vi "LIMITSdll.vi"(8 "error in (no error)":errorcluster, 11 "Inputs":cluster{"htyp":string, "z":dbl[]}) -> (0 "error out":errorcluster, 3 "Outputs":T1)   [LabVIEW 2021]
doc: "subroutine LIMITSdll(htyp, z, tmin, tmax, dmax, pmax, htyp_length)\nReturns limits of a property model as a function of composition. Pure fluid limits were read in from the *.fld files; for mixtures, a simple mole fraction weighting in reduced variables is used.\n\nINPUTS:\nhtyp -- Flag indicating which models are to be checked (character*3) \n ‘EOS’: Equation of state for thermodynamic properties \n ‘ETA’: Viscosity \n ‘TCX’: Thermal conductivity\n ‘STN’: Surface tension\nz -- Composition array (array of mole fractions)\n\nOUTPUTS:\ntmin -- Minimum temperature for model specified by htyp [K]\ntmax -- Maximum temperature [K]\ndmax -- Maximum density [mol/L]\npmax -- Maximum pressure [kPa]\nhtyp_length -- length of variable htyp (default: 3)"
uses:
  REFPROP.dll
panel:
  # "REFPROP-LIMITSdll.vi"
  # "void  LIMITSdll(CStr htyp, double *z, double *tmin, double *tmax, double *dmax, double *pmax, int32_t *hyp_length);"
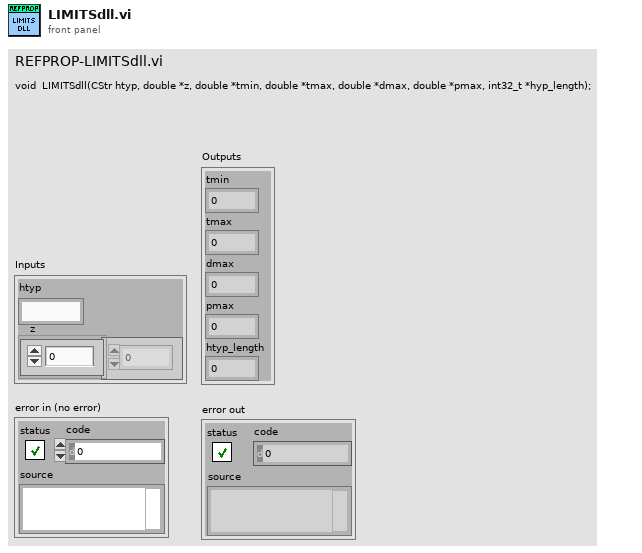
[diagram p1: front panel]
types:
  T1 = cluster{"tmin":dbl, "tmax":dbl, "dmax":dbl, "pmax":dbl, "htyp_length":i32}
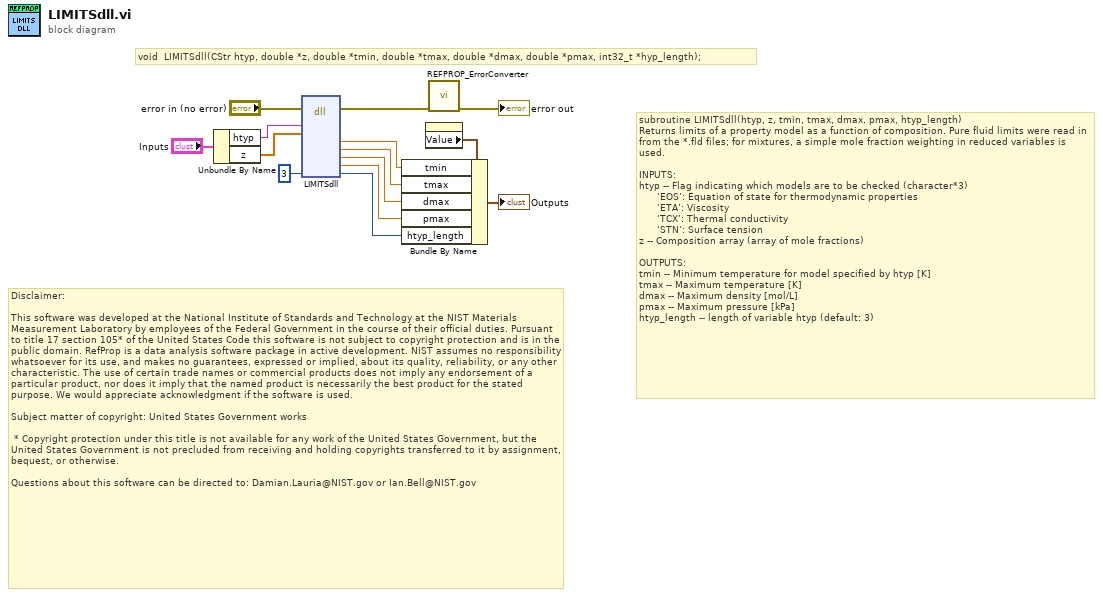
[diagram p0: block diagram]
diagram:
  # "Disclaimer:\n\nThis software was developed at the National Institute of Standards and Technology at the NIST Materials Measurement Laboratory by employees of the Federal Government in the course of their official duties. Pursuant to title 17 section 105* of the United States Code this software is not subject to copyright protection and is in the public domain. RefProp is a data analysis software package in active development. NIST assumes no responsibility whatsoever for its use, and makes no guarantees, expressed or implied, about its quality, reliability, or any other characteristic. The use of certain trade names or commercial products does not imply any endorsement of a particular product, nor does it imply that the named product is necessarily the best product for the stated purpose. We would appreciate acknowledgment if the software is used.\n \nSubject matter of copyright: United States Government works\n  \n * Copyright protection under this title is not available for any work of the United States Government, but the United States Government is not precluded from receiving and holding copyrights transferred to it by assignment, bequest, or otherwise.\n\nQuestions about this software can be directed to: Damian.Lauria@NIST.gov or Ian.Bell@NIST.gov"
  # "void  LIMITSdll(CStr htyp, double *z, double *tmin, double *tmax, double *dmax, double *pmax, int32_t *hyp_length);"
  # "subroutine LIMITSdll(htyp, z, tmin, tmax, dmax, pmax, htyp_length)\nReturns limits of a property model as a function of composition. Pure fluid limits were read in from the *.fld files; for mixtures, a simple mole fraction weighting in reduced variables is used.\n\nINPUTS:\nhtyp -- Flag indicating which models are to be checked (character*3) \n      ‘EOS’: Equation of state for thermodynamic properties \n      ‘ETA’: Viscosity \n      ‘TCX’: Thermal conductivity\n      ‘STN’: Surface tension\nz -- Composition array (array of mole fractions)\n\nOUTPUTS:\ntmin -- Minimum temperature for model specified by htyp [K]\ntmax -- Maximum temperature [K]\ndmax -- Maximum density [mol/L]\npmax -- Maximum pressure [kPa]\nhtyp_length -- length of variable htyp (default: 3)"
  n1 = Unbundle By Name("Inputs") -> ("htyp"=w9:string, "z"=w8:dbl[])
  n2 = dll-call lib="C:/Users/lauria/OneDrive - National Institute of Standards and Technology (NIST)/LabVIEW Projects/7 REFPROP/REFPROP-wrappers-master/REFPROP-wrappers-master/wrappers/Labview/REFPROP/REFPROP.*" fn="LIMITSdll"(error in="error in (no error)", "htyp"=w9, "z"=w8, "hyp_length"=3 ("ln")) -> (error out=w14:errorcluster, "tmin"=w1:dbl, "tmax"=w2:dbl, "dmax"=w3:dbl, "pmax"=w4:dbl, "hyp_length"=w5:i32)  [unwired: 9 in, 1 out]
  n3 = property on="Outputs" class="Clust (strict)"() -> ("Value"=w6:T1)  [unwired: 2 in, 2 out]
  n4 = Bundle By Name(cluster=w6, "tmin"=w1, "tmax"=w2, "dmax"=w3, "pmax"=w4, "htyp_length"=w5) -> (→"Outputs":T1)
  n5 = call "REFPROP_ErrorConverter.vi"("error in (no error)"=w14) -> ("error out"=→"error out":errorcluster)  [unwired: 10 in]
